vi "pre.vi"(5 "A":T1, 9 "B":T1) -> (4 "X 0":bool, 6 "P 1":cluster{"X 1":bool, "X 2":bool, "X 3":bool}, 8 "P 2":T1, 10 "P 3":T1, 15 "P 4":T1)   [LabVIEW 2013]
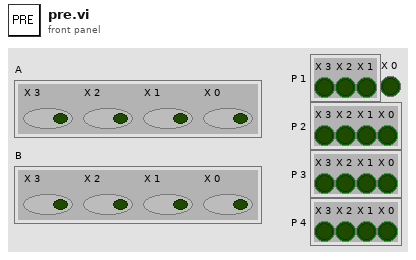
[diagram p1: front panel]
types:
  T1 = cluster{"X 0":bool, "X 1":bool, "X 2":bool, "X 3":bool}
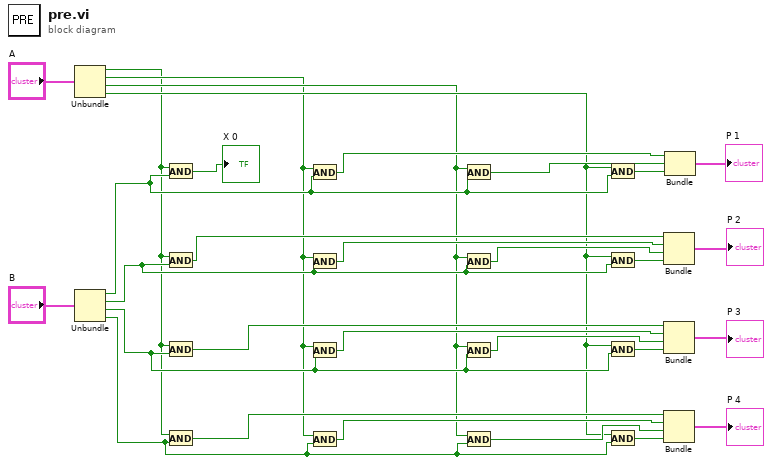
[diagram p0: block diagram]
diagram:
  n1 = Unbundle("A") -> ("X 0"=w2:bool, "X 1"=w3:bool, "X 2"=w4:bool, "X 3"=w5:bool)
  n2 = Unbundle("B") -> ("X 0"=w9:bool, "X 1"=w8:bool, "X 2"=w7:bool, "X 3"=w6:bool)
  n3 = And(x=w2, y=w9) -> (x .and. y?=→"X 0":bool)
  n4 = And(x=w2, y=w8) -> (x .and. y?=w23:bool)
  n5 = And(x=w2, y=w7) -> (x .and. y?=w19:bool)
  n6 = And(x=w2, y=w6) -> (x .and. y?=w15:bool)
  n7 = And(x=w3, y=w9) -> (x .and. y?=w28:bool)
  n8 = And(x=w3, y=w8) -> (x .and. y?=w24:bool)
  n9 = And(x=w3, y=w7) -> (x .and. y?=w20:bool)
  n10 = And(x=w3, y=w6) -> (x .and. y?=w16:bool)
  n11 = And(x=w4, y=w9) -> (x .and. y?=w29:bool)
  n12 = And(x=w4, y=w8) -> (x .and. y?=w25:bool)
  n13 = And(x=w4, y=w7) -> (x .and. y?=w21:bool)
  n14 = And(x=w4, y=w6) -> (x .and. y?=w17:bool)
  n15 = And(x=w5, y=w9) -> (x .and. y?=w30:bool)
  n16 = And(x=w5, y=w8) -> (x .and. y?=w26:bool)
  n17 = And(x=w5, y=w7) -> (x .and. y?=w22:bool)
  n18 = And(x=w5, y=w6) -> (x .and. y?=w18:bool)
  n19 = Bundle(w23, w24, w25, w26) -> (→"P 2":cluster{bool, bool, bool, bool})  [unwired: 1 in]
  n20 = Bundle(w19, w20, w21, w22) -> (→"P 3":cluster{bool, bool, bool, bool})  [unwired: 1 in]
  n21 = Bundle(w15, w16, w17, w18) -> (→"P 4":cluster{bool, bool, bool, bool})  [unwired: 1 in]
  n22 = Bundle(w28, w29, w30) -> (→"P 1":cluster{bool, bool, bool})  [unwired: 1 in]
